vi "CreateInterfaceByID.vi"(8 "error in (no error)":errorcluster, 9 "pInterfaceID":string) -> (0 "error out":errorcluster, 1 "handle":i64 format="%x", 2 "function return":i32 format="%x")   [LabVIEW 2013, in "MvCameraControl.lvlib"]
doc: "MV_CAMCTRL_API int __stdcall MV_CC_CreateInterfaceByID(IN OUT void ** handle, IN const char* pInterfaceID);"
uses:
  MvCameraControl.lvlib
  MvCameraControl.dll
panel:
  out "unsigned byte array":u8[](array[numeric])
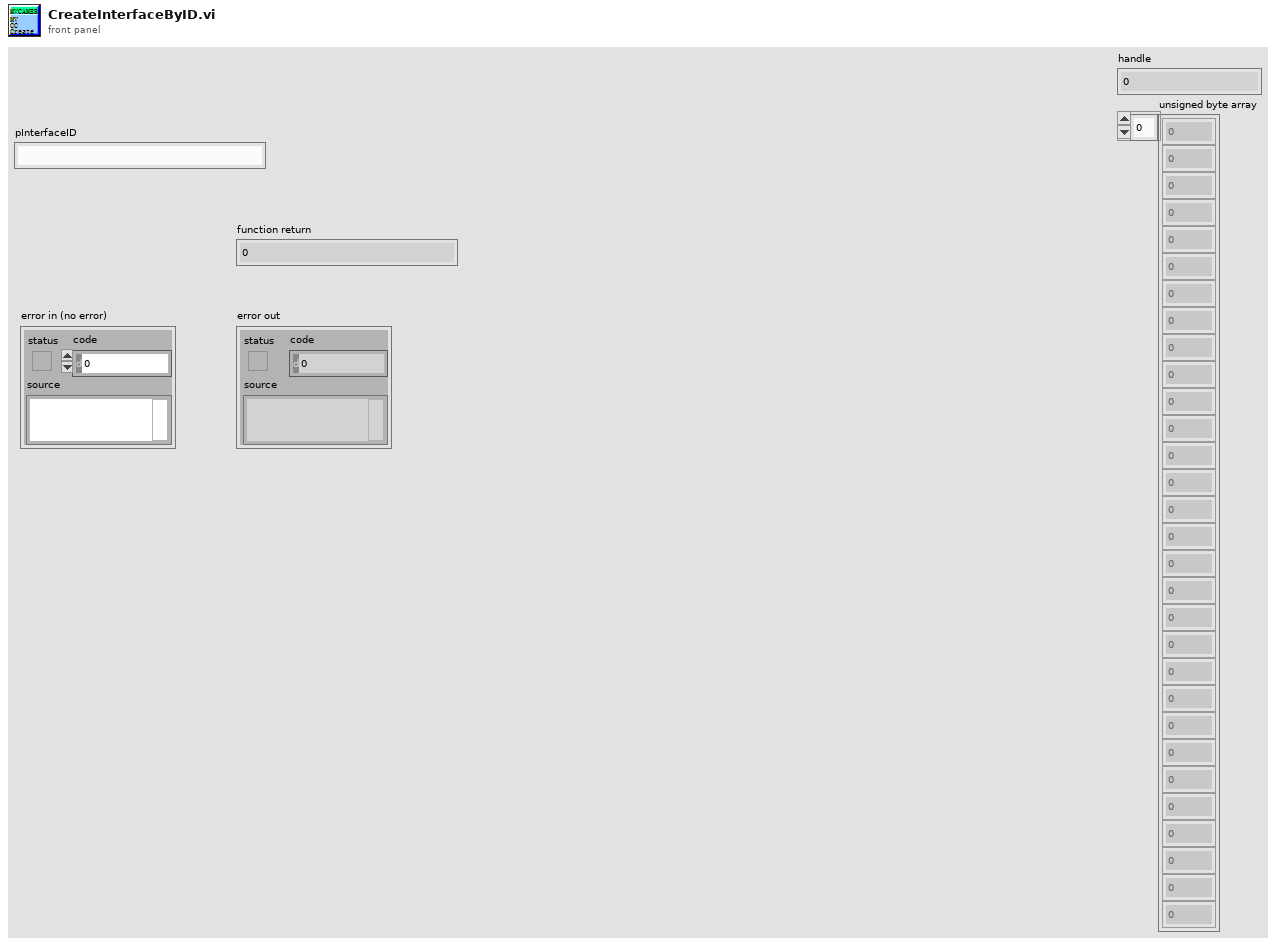
[diagram p1: front panel]
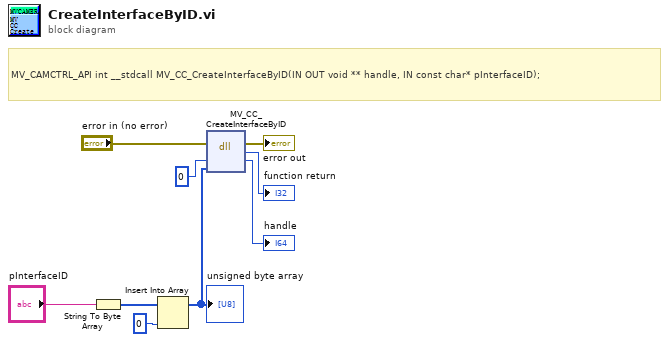
[diagram p0: block diagram]
diagram:
  # "MV_CAMCTRL_API int __stdcall MV_CC_CreateInterfaceByID(IN OUT void ** handle, IN const char* pInterfaceID);"
  n1 = String To Byte Array(string="pInterfaceID") -> (unsigned byte array=w3:u8[])
  n2 = Insert Into Array(array=w3, new element=u8 0 ("new element/subarray")) -> (w1:u8[])  [unwired: 1 in]
  "unsigned byte array" <- w1
  n3 = dll-call lib="MvCameraControl.*" fn="MV_CC_CreateInterfaceByID"(error in="error in (no error)", "handle"=i64 0, "pInterfaceID"=w1) -> (error out=→"error out":errorcluster, "return type"=→"function return":i32, "handle"=→"handle":i64)  [unwired: 3 in, 1 out]
